vi "Pipelined Processing.vi"() -> ()   [LabVIEW 2023]
doc: "The Pipelined Processing example shows how to use feedback nodes to allow different processing functions to operate on different images in the same cycle. This example uses a grab acquisition which works for all camera formats and image sizes. It is recommended to use the Pipelined Processing (Optimized Performance) example if your camera settings work with a ring acquisition.\n\nIn this example, image processing is simulated by a time delay that can be adjusted while the VI is running. When processing is complete, <B>Unlock</B> is called on <B>Image Manager for Grab Acquisition</B> to allow the grab to copy into that image again."
uses:
  SubVIs/Grab Manager Mode.ctl
  <vilib>/vision/driver/IMAQdx.llb/IMAQdx Buffer Number Mode.ctl
  <vilib>/vision/Image Controls.llb/IMAQ Image.ctl
  <vilib>/vision/driver/NI_Vision_Acquisition_Software.lvlib
panel:
  in  "Processing Delay (ms)":dbl=5.0
  out "Image":T1(plugin-control)
  out "Acquired Frame Rate":dbl
  out "Processing Frame Rate":dbl
  in  "Enable Pipelined Processing":bool
  out "Lost Buffer Count":u32
  in  "Number of Images":u32=30
  in  "Camera Name":refnum<k21> caption="IMAQdx Session"
  in  "Stop":bool
  # "Overview: Demonstrates how to process an image using a pipelined approach to improve performance so multiple operations can happen on the same iteration of the loop.\nRequirements: Vision Acquisition Software\nInstructions:\n1. Select the Camera Name\n2. Run the VI and increase the Processing Delay until the Processing Frame Rate is less than the Acquired Frame Rate\n3. Stop the VI and turn on the Enabled Pipelined Processing and repeat step 2 to compare the maximum Processing Delay before falling behind"
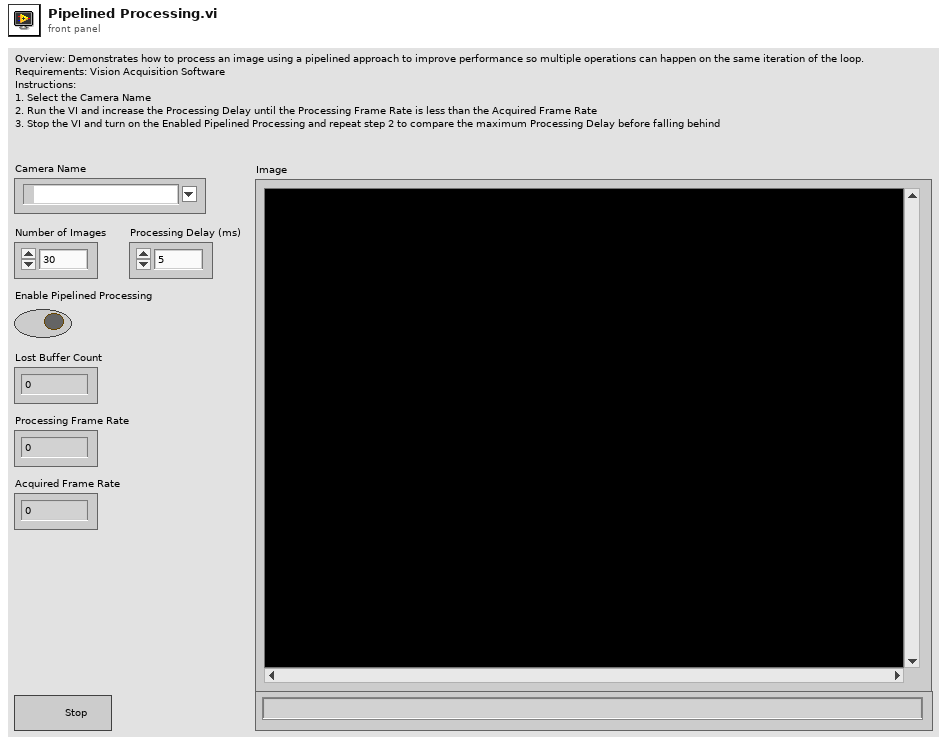
[diagram p1: front panel]
types:
  T1 = typedef "IMAQ Image.ctl" = refnum<image>
  T2 = typedef "Grab Manager Mode.ctl" = enum16{"Create Processing Images", "Lock", "Add Acquired Image", "Get Acquired Image", "Unlock", "Dispose Processing Images"}
  T3 = cluster{"Number of Processing Images":u32, "Image Border Size":u32}
  T4 = typedef "IMAQdx.ctl" = refnum<k21>
  T5 = typedef "NI_Vision_Acquisition_Software.lvlib/IMAQdx Buffer Number Mode.ctl" = enum32{"Next", "Last", "Buffer Number", "Every", "Last New"}
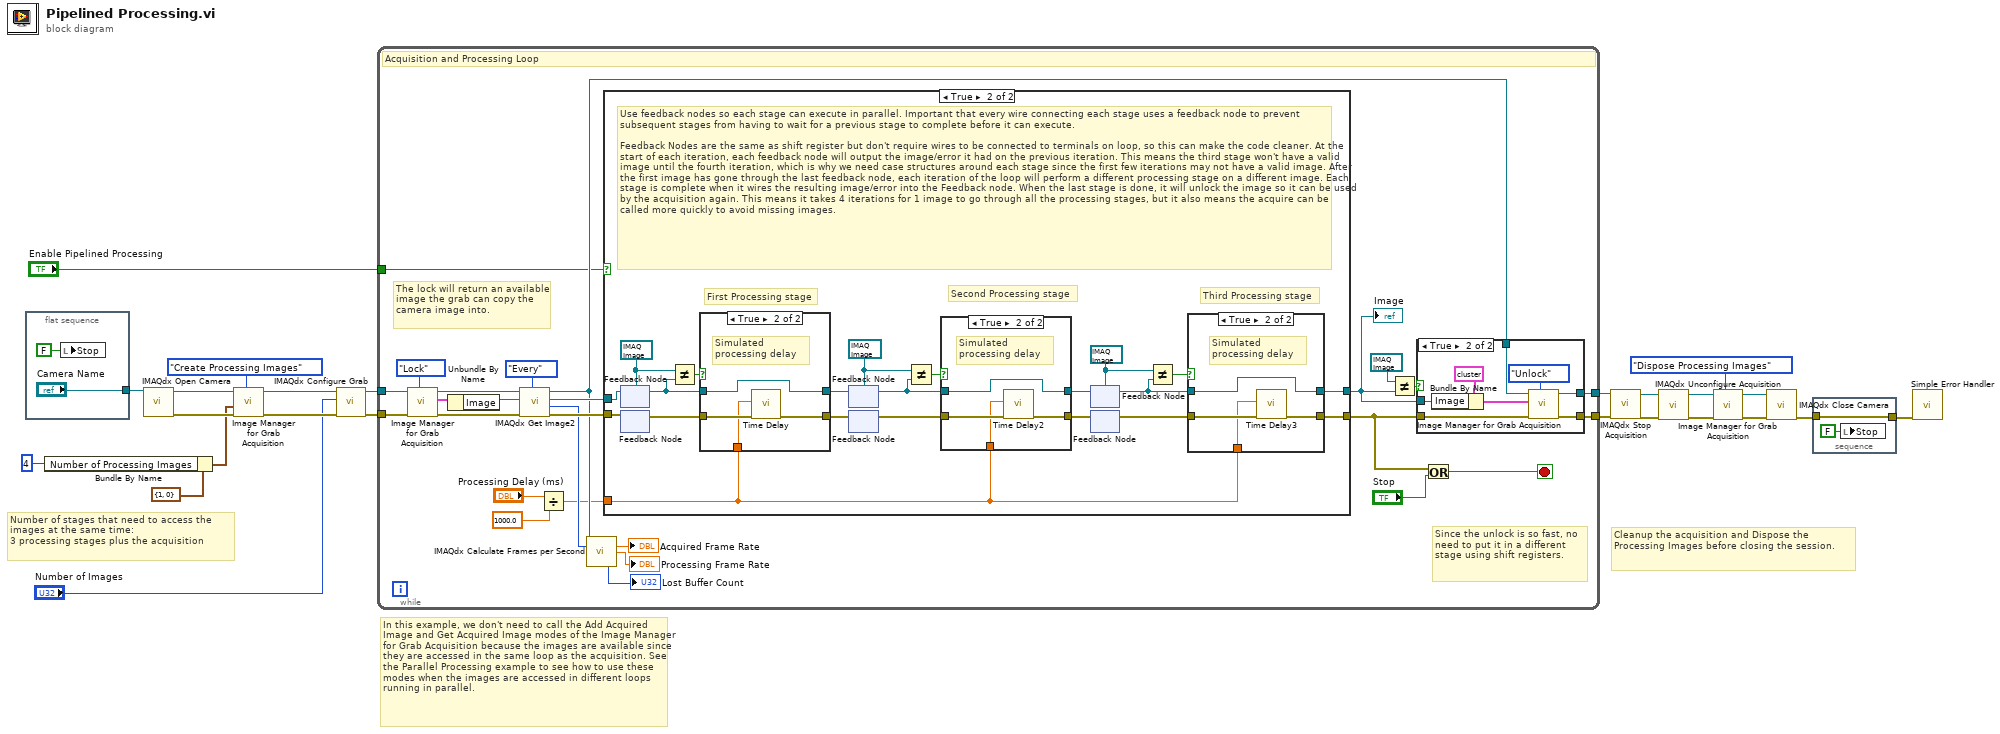
[diagram p0: block diagram]
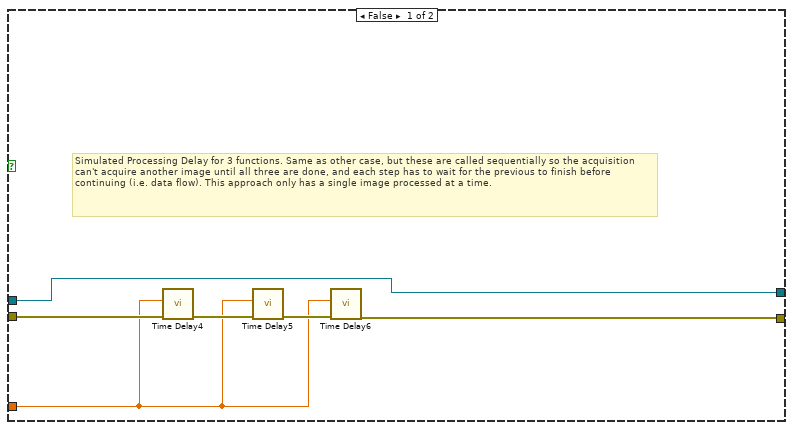
[diagram p2: hidden frame]
diagram:
  # "In this example, we don't need to call the Add Acquired Image and Get Acquired Image modes of the Image Manager for Grab Acquisition because the images are available since they are accessed in the same loop as the acquisition. See the Parallel Processing example to see how to use these modes when the images are accessed in different loops running in parallel."
  # "Number of stages that need to access the images at the same time:\n3 processing stages plus the acquisition"
  # "Cleanup the acquisition and Dispose the Processing Images before closing the session."
  n1 = flat-sequence {
    tunnel: ["Camera Name"] -> w24
    frame #0 {
      n2 = local write "Stop"(FALSE ("Stop")) -> ()
    }
  }
  n3 = Bundle By Name(cluster=T3 {"Number of Processing Images"=1, "Image Border Size"=0} ("Init Settings"), "Number of Processing Images"=u32 4) -> (w13:T3)
  n4 = call <vilib>:"IMAQdx Open Camera.vi"("Session In"=w24) -> ("error out"=w15:errorcluster, "Session Out"=w17:T4)  [unwired: 2 in, 7 out]
  n5 = call "Image Manager for Grab Acquisition.vi"("Mode"=Grab_Manager_Mode."Create Processing Images", "error in (no error)"=w15, "Init Settings"=w13, "Session In"=w17) -> ("error out"=w11:errorcluster, "Session Out"=w12:T4)  [unwired: 4 in, 2 out]
  n6 = call <vilib>:"IMAQdx Configure Grab.vi"("error in"=w11, "Number of Buffers"="Number of Images", "Session In"=w12) -> ("error out"=w8:errorcluster, "Session Out"=w9:T4)  [unwired: 7 in]
  n7 = while {
    tunnel: w8 -> [w31]
    tunnel: w9 -> [w32]
    tunnel: [w45] -> w21
    tunnel: [w46] -> w1
    tunnel: "Enable Pipelined Processing" -> [w39]
    stop <- w40 stop-if-true
    # "The lock will return an available image the grab can copy the camera image into."
    # "Since the unlock is so fast, no need to put it in a different stage using shift registers."
    # "Acquisition and Processing Loop"
    n8 = call "Image Manager for Grab Acquisition.vi"("Mode"=Grab_Manager_Mode."Lock", "error in (no error)"=w31, "Session In"=w32) -> ("error out"=w28:errorcluster, "Image Settings Out"=w29:cluster{"Image":T1, "Buffer Number":u32}, "Session Out"=w30:T4)  [unwired: 5 in, 1 out]
    n9 = Unbundle By Name(w29) -> ("Image"=w27:T1)
    n10 = call <vilib>:"IMAQdx Get Image2.vi"("Buffer Number Mode (Next)"=IMAQdx_Buffer_Number_Mode."Every" ("Buffer Number Mode"), "error in"=w28, "Image In"=w27, "Session In"=w30) -> ("error out"=w51:errorcluster, "Buffer Number Out"=w42:u32, "Image Out"=w50:T1, "Session Out"=w44:T4)  [unwired: 4 in]
    n11 = Divide(x="Processing Delay (ms)", y=1000.0) -> (x/y=w36:dbl)
    n12 = call <vilib>:"IMAQdx Calculate Frames per Second.vi"("Session In"=w44, "Buffer Number"=w42) -> ("Acquired Frames per Second"=→"Acquired Frame Rate":dbl, "Processed Frames per Second"=→"Processing Frame Rate":dbl, "Images Missed"=→"Lost Buffer Count":u32)  [unwired: 7 in, 4 out]
    n13 = case shown="True" w39 {
      tunnel: w51 -> [w59 w80]
      tunnel: w50 -> [w55 w79]
      tunnel: [w56 w78] -> w47
      tunnel: [w55 w64] -> w35
      tunnel: w36 -> [w54 w60]
      frame False {
        # "Simulated Processing Delay for 3 functions. Same as other case, but these are called sequentially so the acquisition can't acquire another image until all three are done, and each step has to wait for the previous to finish before continuing (i.e. data flow). This approach only has a single image processed at a time."
        n14 = call "Time Delay4"("error in (no error)"=w59, "Delay Time (s)"=w54) -> ("error out"=w58:errorcluster)  [unwired: 9 in]
        n15 = call "Time Delay5"("error in (no error)"=w58, "Delay Time (s)"=w54) -> ("error out"=w57:errorcluster)  [unwired: 9 in]
        n16 = call "Time Delay6"("error in (no error)"=w57, "Delay Time (s)"=w54) -> ("error out"=w56:errorcluster)  [unwired: 9 in]
      }
      frame True {
        w61 = T1 refnum ("Image Out")
        w62 = T1 refnum ("Image Out")
        w63 = T1 refnum ("Image Out")
        # "Use feedback nodes so each stage can execute in parallel. Important that every wire connecting each stage uses a feedback node to prevent subsequent stages from having to wait for a previous stage to complete before it can execute.\n\nFeedback Nodes are the same as shift register but don't require wires to be connected to terminals on loop, so this can make the code cleaner. At the start of each iteration, each feedback node will output the image/error it had on the previous iteration. This means the third stage won't have a valid image until the fourth iteration, which is why we need case structures around each stage since the first few iterations may not have a valid image. After the first image has gone through the last feedback node, each iteration of the loop will perform a different processing stage on a different image. Each stage is complete when it wires the resulting image/error into the Feedback node. When the last stage is done, it will unlock the image so it can be used by the acquisition again. This means it takes 4 iterations for 1 image to go through all the processing stages, but it also means the acquire can be called more quickly to avoid missing images."
        # "Third Processing stage"
        # "Second Processing stage"
        # "First Processing stage"
        n17 = feedback #1(w63) -> (w66:T1)
        n18 = feedback-in #1(w79) -> ()
        n19 = feedback #2() -> (w77:errorcluster)  [unwired: 1 in]
        n20 = feedback-in #2(w80) -> ()
        n21 = Not Equal?(x=w63, y=w66) -> (x != y?=w65:bool)
        n22 = case shown="True" w65 {
          tunnel: w77 -> [w93 w98]
          tunnel: w66 -> [w94 w95]
          tunnel: [w94 w95] -> w76
          tunnel: [w93 w97] -> w75
          tunnel: w60 -> [_ w96]
          frame False {
            # "No image to process"
          }
          frame True {
            # "Simulated processing delay"
            n23 = call "Time Delay"("error in (no error)"=w98, "Delay Time (s)"=w96) -> ("error out"=w97:errorcluster)  [unwired: 9 in]
          }
        }
        n24 = feedback #3(w62) -> (w73:T1)
        n25 = feedback-in #3(w76) -> ()
        n26 = feedback #4() -> (w72:errorcluster)  [unwired: 1 in]
        n27 = feedback-in #4(w75) -> ()
        n28 = Not Equal?(x=w62, y=w73) -> (x != y?=w74:bool)
        n29 = case shown="True" w74 {
          tunnel: w72 -> [w87 w92]
          tunnel: w73 -> [w88 w89]
          tunnel: [w88 w89] -> w71
          tunnel: [w87 w91] -> w70
          tunnel: w60 -> [_ w90]
          frame False {
            # "No image to process"
          }
          frame True {
            # "Simulated processing delay"
            n30 = call "Time Delay2"("error in (no error)"=w92, "Delay Time (s)"=w90) -> ("error out"=w91:errorcluster)  [unwired: 9 in]
          }
        }
        n31 = feedback #5(w61) -> (w69:T1)
        n32 = feedback-in #5(w71) -> ()
        n33 = feedback #6() -> (w68:errorcluster)  [unwired: 1 in]
        n34 = feedback-in #6(w70) -> ()
        n35 = Not Equal?(x=w61, y=w69) -> (x != y?=w67:bool)
        n36 = case shown="True" w67 {
          tunnel: w68 -> [w81 w86]
          tunnel: w69 -> [w82 w83]
          tunnel: [w82 w83] -> w64
          tunnel: [w81 w85] -> w78
          tunnel: w60 -> [_ w84]
          frame False {
            # "No image to process"
          }
          frame True {
            # "Simulated processing delay"
            n37 = call "Time Delay3"("error in (no error)"=w86, "Delay Time (s)"=w84) -> ("error out"=w85:errorcluster)  [unwired: 9 in]
          }
        }
      }
    }
    "Image" <- w35
    n38 = Not Equal?(x=T1 refnum ("Image Out"), y=w35) -> (x != y?=w43:bool)
    n39 = case shown="True" w43 {
      tunnel: w47 -> [w100 w107]
      tunnel: [w100 w106] -> w46
      tunnel: [w99 w105] -> w45
      tunnel: w44 -> [w99 w104]
      tunnel: w35 -> [_ w102]
      frame False {
      }
      frame True {
        n40 = Bundle By Name(cluster=cluster{"Image":T1, "Buffer Number":u32} {"Image"=refnum, "Buffer Number"=0} ("Image Settings In"), "Image"=w102) -> (w101:cluster{"Image":T1, "Buffer Number":u32})
        n41 = call "Image Manager for Grab Acquisition.vi"("Mode"=Grab_Manager_Mode."Unlock", "error in (no error)"=w107, "Image Settings In"=w101, "Session In"=w104) -> ("error out"=w106:errorcluster, "Session Out"=w105:T4)  [unwired: 4 in, 2 out]
      }
    }
    n42 = Or(x=w47, y="Stop") -> (x .or. y?=w40:bool)
  }
  n43 = call <vilib>:"IMAQdx Stop Acquisition.vi"("error in"=w1, "Session In"=w21) -> ("error out"=w22:errorcluster, "Session Out"=w23:T4)  [unwired: 8 out]
  n44 = call <vilib>:"IMAQdx Unconfigure Acquisition.vi"("error in"=w22, "Session In"=w23) -> ("error out"=w5:errorcluster, "Session Out"=w6:T4)  [unwired: 8 out]
  n45 = call "Image Manager for Grab Acquisition.vi"("Mode"=Grab_Manager_Mode."Dispose Processing Images", "error in (no error)"=w5, "Session In"=w6) -> ("error out"=w3:errorcluster, "Session Out"=w4:T4)  [unwired: 5 in, 2 out]
  n46 = call <vilib>:"IMAQdx Close Camera.vi"("error in"=w3, "Session In"=w4) -> ("error out"=w2:errorcluster)  [unwired: 9 out]
  n47 = stacked-sequence {
    tunnel: [w109] -> w20
    tunnel: w2 -> [w109]
    frame #0 {
      n48 = local write "Stop"(FALSE ("Stop")) -> ()
    }
  }
  n49 = call <vilib>:"Simple Error Handler.vi"("error in (no error)"=w20) -> ()  [unwired: 4 in, 5 out]
